vi "Render.vi"(8 "error in (no error)":errorcluster, 11 "Test_Button in":refnum<class "Test_Button.lvclass">) -> (0 "error out":errorcluster)   [LabVIEW 2020, in "Test_Button.lvclass"]
uses:
  Test_Button.lvclass
  Test_Button.lvclass/Test_Button.ctl
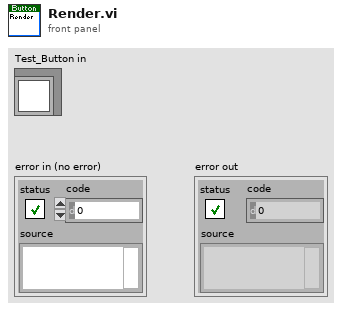
[diagram p1: front panel]
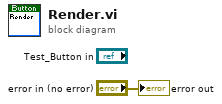
[diagram p0: block diagram]
diagram:
  "error out" <- "error in (no error)"
